vi "Write QuotesOnTableName.vi"(8 "error in (no error)":errorcluster, 10 "QuotesOnTableName":bool, 11 "SqliteConnection in":refnum<class "DBC.lvclass">) -> (0 "error out":errorcluster, 3 "SqliteConnection out":refnum<class "DBC.lvclass">)   [LabVIEW 2020, in "ORM_DBC_Sqlite.lvlib" / "DBC.lvclass"]
uses:
  DBC.lvclass
  DBC.lvclass/DBC.ctl
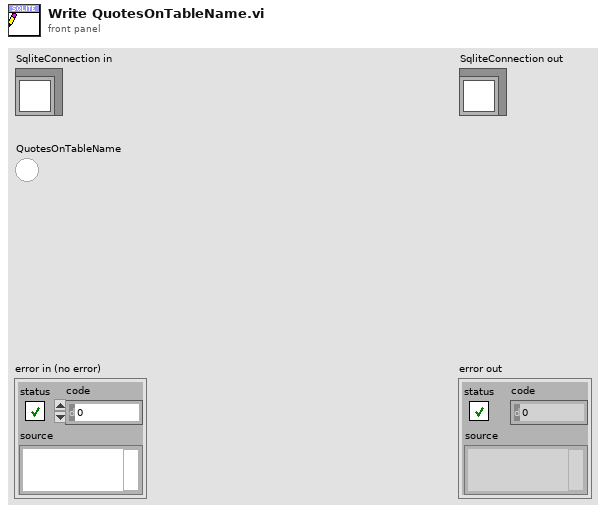
[diagram p1: front panel]
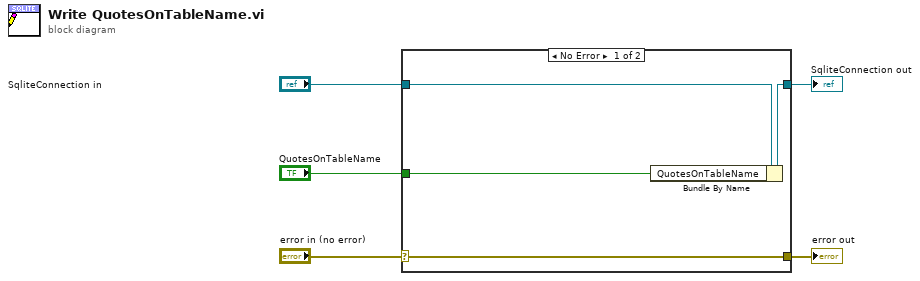
[diagram p0: block diagram]
diagram:
  n1 = case shown="No Error" "error in (no error)" {
    selector: "error in (no error)" -> [w9 w10]
    tunnel: [w9 w10] -> w4
    tunnel: [w7 w11] -> w2
    tunnel: "SqliteConnection in" -> [w8 w11]
    tunnel: "QuotesOnTableName" -> [w6 _]
    frame No Error {
      n2 = Bundle By Name(cluster=w8, "QuotesOnTableName"=w6) -> (w7:refnum<class "DBC.lvclass">)
    }
    frame Error {
    }
  }
  "error out" <- w4
  "SqliteConnection out" <- w2
